vi "set_relay.vi"(6 "ch_4":bool, 8 "ch_3":bool, 9 "ch_2":bool, 10 "ch_1":bool, 11 "Handle":u64) -> (0 "message":string, 1 "ch_2_out":bool, 2 "ch_1_out":bool, 3 "Handle_out":u64, 4 "status":bool)   [LabVIEW 2019]
panel:
  out "bytes_wait":u32
  out "bytes_written":u32
  out "status_read":u32(ring) items=["FT_OK", "FT_INVALID_HANDLE", "FT_DEVICE_NOT_FOUND", "FT_DEVICE_NOT_OPENED", "FT_IO_ERROR", "FT_INSUFFICIENT_RESOURCES", "FT_INVALID_PARAMETER", "FT_INVALID_BAUD_RATE", "FT_DEVICE_NOT_OPENED_FOR_ERASE", "FT_DEVICE_NOT_OPENED_FOR_WRITE", "FT_FAILED_TO_WRITE_DEVICE", "FT_EEPROM_READ_FAILED", "FT_EEPROM_WRITE_FAILED", "FT_EEPROM_ERASE_FAILED", "FT_EEPROM_NOT_PRESENT", "FT_EEPROM_NOT_PROGRAMMED", "FT_INVALID_ARGS", "FT_NOT_SUPPORTED", "FT_OTHER_ERROR"]
  out "status_write":u32(ring) items=["FT_OK", "FT_INVALID_HANDLE", "FT_DEVICE_NOT_FOUND", "FT_DEVICE_NOT_OPENED", "FT_IO_ERROR", "FT_INSUFFICIENT_RESOURCES", "FT_INVALID_PARAMETER", "FT_INVALID_BAUD_RATE", "FT_DEVICE_NOT_OPENED_FOR_ERASE", "FT_DEVICE_NOT_OPENED_FOR_WRITE", "FT_FAILED_TO_WRITE_DEVICE", "FT_EEPROM_READ_FAILED", "FT_EEPROM_WRITE_FAILED", "FT_EEPROM_ERASE_FAILED", "FT_EEPROM_NOT_PRESENT", "FT_EEPROM_NOT_PROGRAMMED", "FT_INVALID_ARGS", "FT_NOT_SUPPORTED", "FT_OTHER_ERROR"]
  out "string_write":string
  out "channel_bits":u8=1 max=15
  out "string_read":string
  out "bytes_read":u32
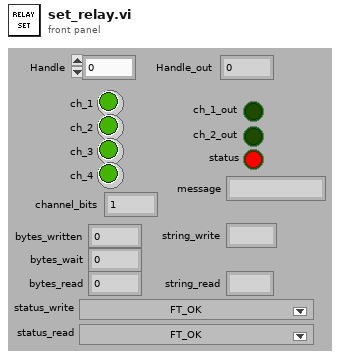
[diagram p1: front panel]
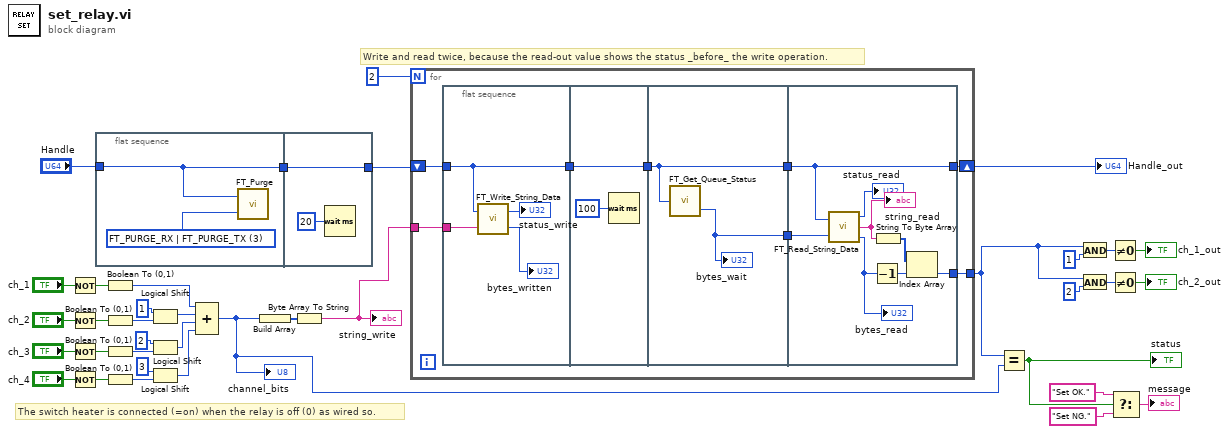
[diagram p0: block diagram]
diagram:
  # "The switch heater is connected (=on) when the relay is off (0) as wired so."
  # "Write and read twice, because the read-out value shows the status _before_ the write operation."
  n1 = Not(x="ch_1") -> (.not. x?=w4:bool)
  n2 = Not(x="ch_2") -> (.not. x?=w3:bool)
  n3 = Not(x="ch_3") -> (.not. x?=w2:bool)
  n4 = Not(x="ch_4") -> (.not. x?=w1:bool)
  n5 = flat-sequence {
    tunnel: "Handle" -> [w38]
    tunnel: [w38] -> w12
    tunnel: w12 -> [w40]
    tunnel: [w40] -> w11
    frame #0 {
      w39 = u32 3 items=["FT_PURGE_RX"=1, "FT_PURGE_TX"=2, "FT_PURGE_RX | FT_PURGE_TX"=3] ("Purge Flags")
      n6 = call "FT_Purge.vi"("Purge Flags"=w39, "Handle"=w38) -> ()  [unwired: 1 out]
    }
    frame #1 {
      n7 = Wait (ms)(milliseconds to wait=u32 20) -> ()  [unwired: 1 out]
    }
  }
  n8 = Boolean To (0,1)(Boolean=w4) -> (0, 1=w27:i16)
  n9 = Boolean To (0,1)(Boolean=w3) -> (0, 1=w33:i16)
  n10 = Boolean To (0,1)(Boolean=w2) -> (0, 1=w31:i16)
  n11 = Boolean To (0,1)(Boolean=w1) -> (0, 1=w30:i16)
  n12 = Logical Shift(y=i16 1, x=w33) -> (x << y=w26:i16)
  n13 = Logical Shift(y=i16 2, x=w31) -> (x << y=w25:i16)
  n14 = Logical Shift(y=i16 3, x=w30) -> (x << y=w24:i16)
  n15 = Compound Arithmetic op=ADD(w27, w26, w25, w24) -> (w9:i16)
  "channel_bits" <- w9
  n16 = Build Array(w9) -> (w23:i16[])
  n17 = Byte Array To String(unsigned byte array=w23) -> (string=w20:string)
  "string_write" <- w20
  n18 = for {
    N: 2 -> [_]
    tunnel: w20 -> [w47]
    shift-right: [w46] -> w21
    shift-left: w11 -> [w48]
    tunnel: [w42] -> w10
    n19 = flat-sequence {
      tunnel: w48 -> [w51]
      tunnel: w47 -> [w52]
      tunnel: [w51] -> w49
      tunnel: [w54] -> w45
      tunnel: w49 -> [w54]
      tunnel: w45 -> [w57]
      tunnel: [w57] -> w44
      tunnel: [w56] -> w43
      tunnel: w44 -> [w64]
      tunnel: [w64] -> w46
      tunnel: w43 -> [w63]
      tunnel: [w58] -> w42
      frame #0 {
        n20 = call "FT_Write_String_Data.vi"("Buffer"=w52, "Handle"=w51) -> ("Bytes Written"=→"bytes_written":u32, "FT_Status"=→"status_write":u32)
      }
      frame #1 {
        n21 = Wait (ms)(milliseconds to wait=u32 100) -> ()  [unwired: 1 out]
      }
      frame #2 {
        n22 = call "FT_Get_Queue_Status.vi"("Handle"=w57) -> ("Bytes Waiting"=w56:u32)  [unwired: 1 out]
        "bytes_wait" <- w56
      }
      frame #3 {
        n23 = call "FT_Read_String_Data.vi"("Handle"=w64, "Bytes To Read"=w63) -> ("FT_Status"=→"status_read":u32, "Read Data"=w62:string, "Bytes Read"=w59:u32)
        "bytes_read" <- w59
        "string_read" <- w62
        n24 = Decrement(x=w59) -> (x-1=w60:u32)
        n25 = String To Byte Array(string=w62) -> (unsigned byte array=w61:u8[])
        n26 = Index Array(array=w61, index=w60) -> (element=w58:u8)
      }
    }
  }
  "Handle_out" <- w21
  n27 = Equal?(x=w10, y=w9) -> (x = y?=w8:bool)
  "status" <- w8
  n28 = And(x=w10, y=u32 1) -> (x .and. y?=w18:u32)
  n29 = And(x=w10, y=u32 2) -> (x .and. y?=w15:u32)
  n30 = Not Equal To 0?(x=w18) -> (x != 0?=→"ch_1_out":bool)
  n31 = Not Equal To 0?(x=w15) -> (x != 0?=→"ch_2_out":bool)
  n32 = Select(t="Set OK." ("message"), s=w8, f="Set NG." ("message")) -> (s? t:f=→"message":string)
